vi "section_parameters_cluster_from_writeable_section_parameters_cluster.vi"(8 "Error In":errorcluster, 11 "Writeable Parameters":T1) -> (0 "Error Out":errorcluster, 3 "Section Parameters":T2)   [LabVIEW 2019]
doc: "Convert from the writeable cluster to the real section parameters cluster with enums and paths."
uses:
  section_parameters_cluster_typedef.ctl
  sections_method_enum_typedef.ctl
  sections_edge_mode_enum_typedef.ctl
  sections_roi_size_enum_typedef.ctl
  xi_angles_enum_typedef.ctl
  writeable_section_parameters_cluster_typedef.ctl
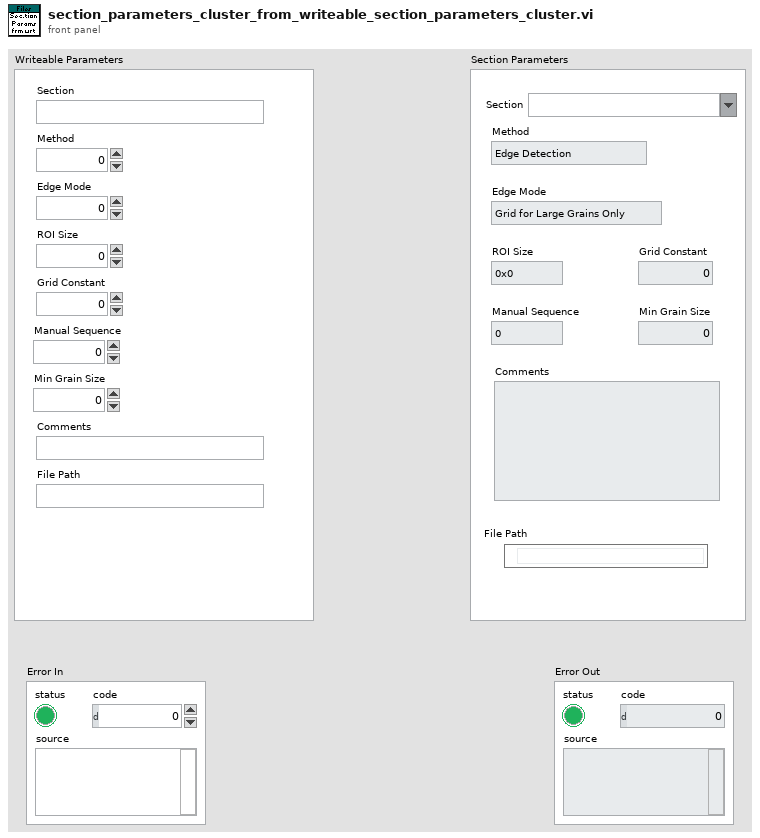
[diagram p1: front panel]
types:
  T1 = typedef "writeable_section_parameters_cluster_typedef.ctl" = cluster{"Section":string, "Method":i32, "Edge Mode":i32, "Grid Constant":i32, "Manual Sequence":i32, "ROI Size":i32, "Min Grain Size":dbl, "Comments":string, "File Path":string}
  T2 = typedef "section_parameters_cluster_typedef.ctl" = cluster{"Section":string, "Method":T3, "Edge Mode":T4, "ROI Size":T5, "Manual Sequence":T6, "Grid Constant":i32, "Min Grain Size":dbl, "Comments":string, "File Path":path}
  T3 = typedef "sections_method_enum_typedef.ctl" = enum16{"Edge Detection", "Grid Only", "Manual Selection", "Existing Edges"}
  T4 = typedef "sections_edge_mode_enum_typedef.ctl" = enum16{"Grid for Large Grains Only", "Grid", "No Grid"}
  T5 = typedef "sections_roi_size_enum_typedef.ctl" = enum16{"0x0", "1x1", "2x2", "3x3", "4x4", "5x5", "6x6"}
  T6 = typedef "xi_angles_enum_typedef.ctl" = enum16{"0", "45"}
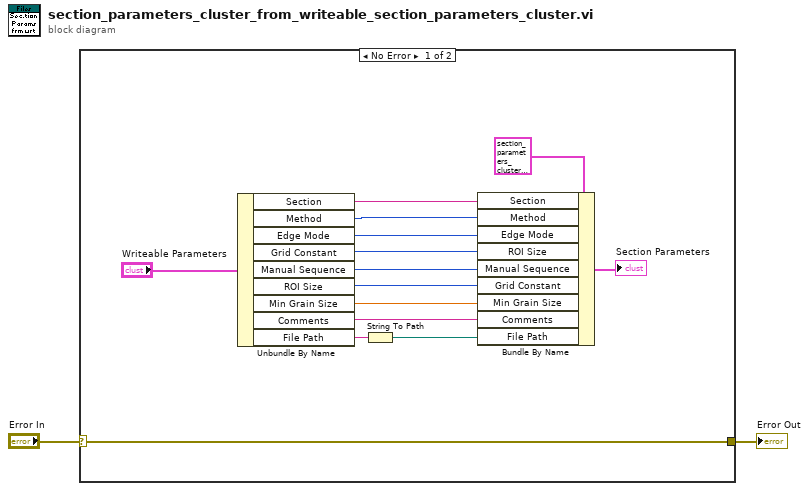
[diagram p0: block diagram]
diagram:
  n1 = case shown="No Error" "Error In" {
    selector: "Error In" -> [w16 w17]
    tunnel: [w16 w17] -> w1
    frame No Error {
      n2 = Unbundle By Name("Writeable Parameters") -> ("Section"=w3:string, "Method"=w4:i32, "Edge Mode"=w5:i32, "Grid Constant"=w6:i32, "Manual Sequence"=w7:i32, "ROI Size"=w8:i32, "Min Grain Size"=w9:dbl, "Comments"=w10:string, "File Path"=w14:string)
      n3 = String To Path(string=w14) -> (path=w11:path)
      n4 = Bundle By Name(cluster=T2 {"Section"="", "Method"=enum."Edge Detection", "Edge Mode"=enum."Grid for Large Grains Only", "ROI Size"=enum."0x0", "Manual Sequence"=enum."0", "Grid Constant"=0, "Min Grain Size"=0.0, "Comments"="", "File Path"=path ""} ("Section Parameters"), "Section"=w3, "Method"=w4, "Edge Mode"=w5, "ROI Size"=w6, "Manual Sequence"=w7, "Grid Constant"=w8, "Min Grain Size"=w9, "Comments"=w10, "File Path"=w11) -> (→"Section Parameters":T2)
    }
    frame Error {
    }
  }
  "Error Out" <- w1
